vi "Camera.vi"(11 "Refnum in":T2) -> (0 "error out":errorcluster)   [LabVIEW 2015]
uses:
  <vilib>/userdefined/High Color/IMAQdx.ctl
  <vilib>/vision/driver/NI_Vision_Acquisition_Software.lvlib
panel:
  in  "Stop Button":bool
  out "Image":T1(plugin-control)
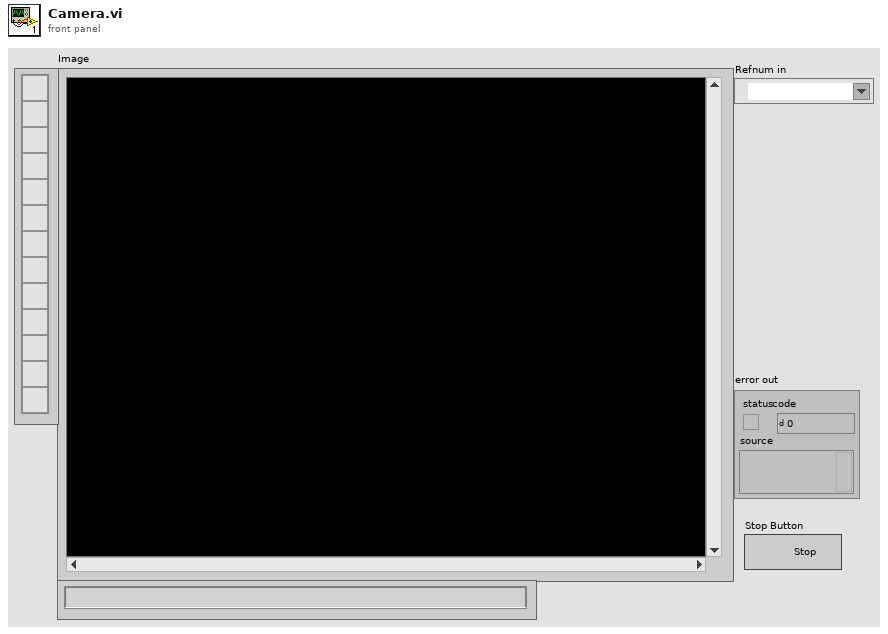
[diagram p1: front panel]
types:
  T1 = typedef "IMAQ Image.ctl" = refnum<image>
  T2 = typedef "IMAQdx.ctl" = refnum<k21>
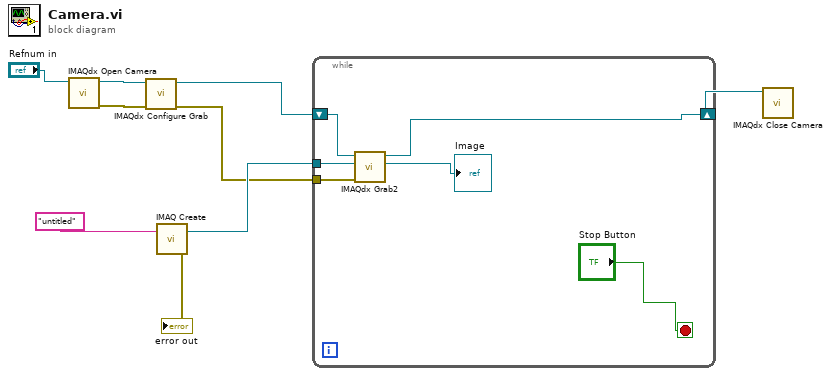
[diagram p0: block diagram]
diagram:
  n1 = call <vilib>:"IMAQdx Open Camera.vi"("Session In"="Refnum in") -> ("error out"=w4:errorcluster, "Session Out"=w3:T2)  [unwired: 9 in]
  n2 = call <vilib>:"IMAQdx Configure Grab.vi"("error in"=w4, "Session In"=w3) -> ("error out"=w5:errorcluster, "Session Out"=w6:T2)  [unwired: 8 in]
  n3 = call "IMAQ Create"("Image Name"="untitled") -> ("New Image"=w7:T1, "error out"=→"error out":errorcluster)  [unwired: 4 in]
  n4 = while {
    tunnel: w7 -> [w15]
    tunnel: w5 -> [w13]
    shift-right: [w11] -> w1
    shift-left: w6 -> [w14]
    stop <- "Stop Button" stop-if-true
    n5 = call <vilib>:"IMAQdx Grab2.vi"("error in"=w13, "Image In"=w15, "Session In"=w14) -> ("Image Out"=→"Image":T1, "Session Out"=w11:T2)  [unwired: 5 in, 2 out]
  }
  n6 = call <vilib>:"IMAQdx Close Camera.vi"("Session In"=w1) -> ()  [unwired: 10 in, 1 out]
